vi "Helper SubVI - Extract Heart Rate.vi"(6 "threshold":dbl=0.6, 9 "last peak":dbl, 10 "trend":cluster{"locations":dbl[], "amplitudes":dbl[]}, 11 "peaks":cluster{"locations":dbl[], "amplitudes":dbl[]}) -> (4 "last peak out":dbl, 5 "HR":dbl[](array[numeric]))   [LabVIEW 2023]
doc: "Extracts the heart rate."
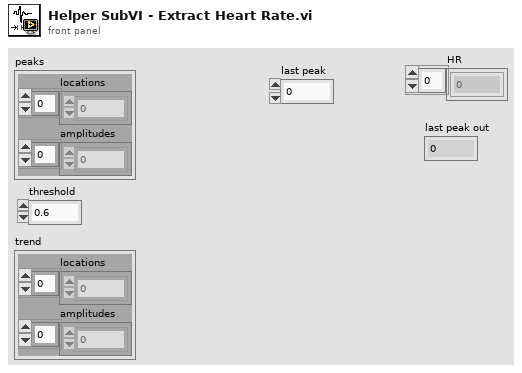
[diagram p1: front panel]
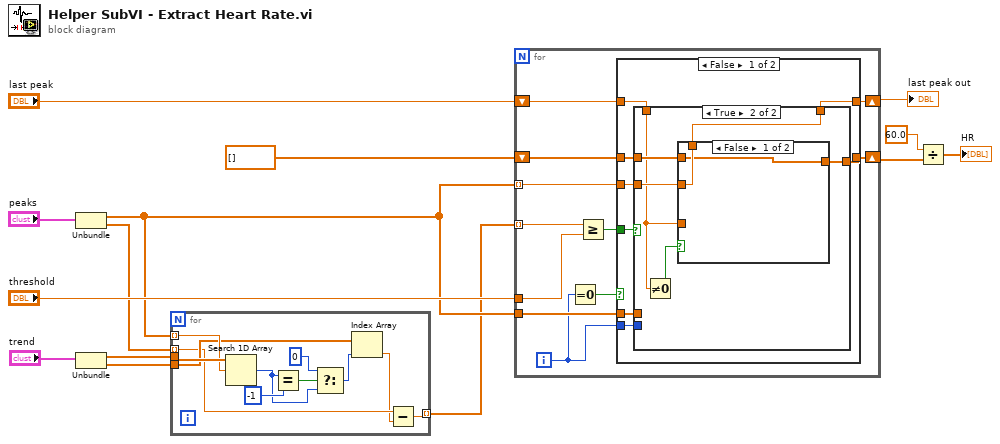
[diagram p0: block diagram]
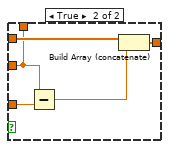
[diagram p3: hidden frame]
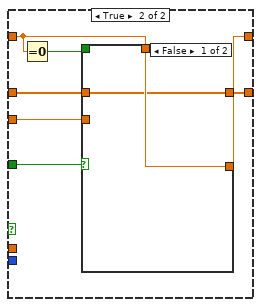
[diagram p4: hidden frame]
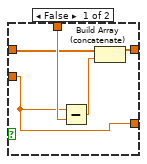
[diagram p6: hidden frame]
diagram:
  n1 = Unbundle("peaks") -> ("locations"=w6:dbl[], "amplitudes"=w5:dbl[])
  n2 = Unbundle("trend") -> ("locations"=w3:dbl[], "amplitudes"=w2:dbl[])
  n3 = for {
    tunnel: w6 -> [w24] mode=indexing
    tunnel: w5 -> [w17] mode=indexing
    tunnel: w3 -> [w25]
    tunnel: w2 -> [w19]
    tunnel: [w15] -> w1 mode=indexing
    n4 = Search 1D Array(1D array=w25, element=w24) -> (index of element=w20:i32)  [unwired: 1 out]
    n5 = Equal?(x=w20, y=-1) -> (x = y?=w22:bool)
    n6 = Select(t=0 ("y"), s=w22, f=w20) -> (s? t:f=w18:i32)
    n7 = Index Array(array=w19, index=w18) -> (element=w16:dbl)
    n8 = Subtract(x=w17, y=w16) -> (x-y=w15:dbl)
  }
  n9 = for {
    tunnel: w6 -> [w27] mode=indexing
    tunnel: w1 -> [w36] mode=indexing
    tunnel: "threshold" -> [w35]
    shift-right: [w33] -> w9
    shift-left: dbl[] [] -> [w32]
    tunnel: w6 -> [w31]
    shift-right: [w26] -> w7
    shift-left: "last peak" -> [w28]
    i -> [w30]
    n10 = Equal To 0?(x=w30) -> (x = 0?=w29:bool)
    n11 = Greater Or Equal?(x=w36, y=w35) -> (x >= y?=w34:bool)
    n12 = case shown="False" w29 {
      tunnel: w34 -> [w44 w60]
      tunnel: w27 -> [w43 w63]
      tunnel: [w42 w64] -> w33
      tunnel: w32 -> [w41 w65]
      tunnel: w31 -> [w40 _]
      tunnel: w30 -> [w39 _]
      tunnel: w28 -> [w38 w62]
      tunnel: [w37 w61] -> w26
      frame False {
        n13 = case shown="True" w44 {
          tunnel: w43 -> [_ w50]
          tunnel: [w46 w52] -> w42
          tunnel: w41 -> [w46 w51]
          tunnel: w40 -> [_ _]
          tunnel: w39 -> [_ _]
          tunnel: w38 -> [w45 w49]
          tunnel: [w45 w47] -> w37
          frame False {
          }
          frame True {
            n14 = Not Equal To 0?(x=w49) -> (x != 0?=w48:bool)
            n15 = case shown="False" w48 {
              tunnel: [w53 w59] -> w52
              tunnel: w51 -> [w53 w58]
              tunnel: w50 -> [w54 w55]
              tunnel: w49 -> [_ w56]
              tunnel: [w54 w55] -> w47
              frame False {
              }
              frame True {
                n16 = Subtract(x=w55, y=w56) -> (x-y=w57:dbl)
                n17 = Build Array (concatenate)(w58, w57) -> (w59:dbl[])
              }
            }
          }
        }
      }
      frame True {
        n18 = Equal To 0?(x=w62) -> (x = 0?=w66:bool)
        n19 = case shown="False" w60 {
          tunnel: w66 -> [_ w74]
          tunnel: w65 -> [w67 w73]
          tunnel: [w67 w72] -> w64
          tunnel: w63 -> [_ w71]
          tunnel: w62 -> [w68 w70]
          tunnel: [w68 w69] -> w61
          frame False {
          }
          frame True {
            n20 = case shown="True" w74 {
              tunnel: w73 -> [w78 w81]
              tunnel: [w76 w81] -> w72
              tunnel: w71 -> [w75 w80]
              tunnel: w70 -> [w79 _]
              tunnel: [w75 w80] -> w69
              frame False {
                n21 = Subtract(x=w75, y=w79) -> (x-y=w77:dbl)
                n22 = Build Array (concatenate)(w78, w77) -> (w76:dbl[])
              }
              frame True {
              }
            }
          }
        }
      }
    }
  }
  "last peak out" <- w7
  n23 = Divide(x=60.0, y=w9) -> (x/y=→"HR":dbl[])
